vi "NanotecSMCPDDriver.get status.vi"(0 "VISA resource name":refnum<visa-resource-name>, 1 "contollerID":i32=-1, 5 "error in (no error)":errorcluster) -> (14 "VISA resource name out":refnum<visa-resource-name>, 15 "contollerID out":i32=-1, 17 "actStatus":T1, 19 "error out":errorcluster)   [LabVIEW 2015, in "NanotecSMCPDDriver.lvlib"]
doc: "Gets the status of the controller."
uses:
  NanotecSMCPDDriver.lvlib
  NanotecSMCPDDriver.status type.ctl
panel:
  in  "actStatus type":T1
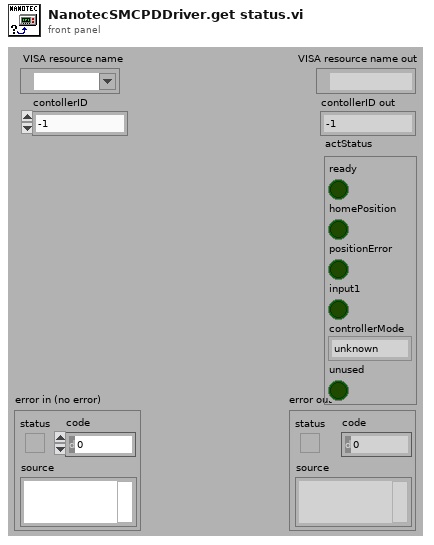
[diagram p1: front panel]
types:
  T1 = typedef "NanotecSMCPDDriver.lvlib/NanotecSMCPDDriver.status type.ctl" = cluster{"ready":bool, "homePosition":bool, "positionError":bool, "input1":bool, "controllerMode":enum16{"unknown", "position", "speed", "flagPosition", "clockDirection", "analog", "joystick", "unused"}, "unused":bool}
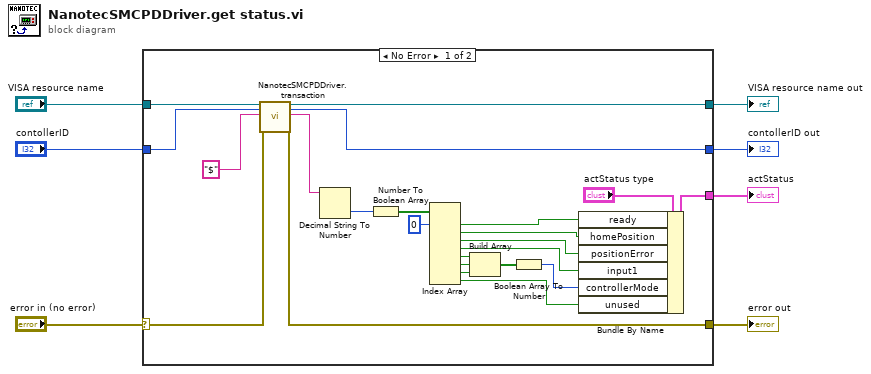
[diagram p0: block diagram]
diagram:
  n1 = case shown="No Error" "error in (no error)" {
    selector: "error in (no error)" -> [w23 w31]
    tunnel: [w26 w33] -> w7
    tunnel: [w24 w31] -> w6
    tunnel: "VISA resource name" -> [w30 w33]
    tunnel: "contollerID" -> [w28 w32]
    tunnel: [w27 w32] -> w3
    tunnel: [w8 _] -> w1
    frame No Error {
      n2 = call "NanotecSMCPDDriver.transaction.vi"("VISAresource"=w30, "contollerID"=w28, "commandString"="$", "error in (no error)"=w23) -> ("VISAresource out"=w26:refnum<visa-resource-name>, "contollerID out"=w27:i32, "response"=w25:string, "error out"=w24:errorcluster)  [unwired: 10 in, 2 out]
      n3 = Decimal String To Number(string=w25) -> (number=w22:i32)  [unwired: 2 in, 1 out]
      n4 = Number To Boolean Array(number=w22) -> (Boolean array=w21:bool[])
      n5 = Index Array(array=w21, index #1=0 ("index")) -> (element #1=w18:bool, element #2=w17:bool, element #3=w16:bool, element #4=w15:bool, element #5=w14:bool, element #6=w13:bool, element #7=w12:bool, element #8=w9:bool)  [unwired: 7 in]
      n6 = Build Array(w14, w13, w12) -> (w11:bool[])
      n7 = Boolean Array To Number(Boolean array=w11) -> (number=w10:u32)
      n8 = Bundle By Name(cluster="actStatus type", "ready"=w18, "homePosition"=w17, "positionError"=w16, "input1"=w15, "controllerMode"=w10, "unused"=w9) -> (w8:T1)
    }
    frame Error {
    }
  }
  "VISA resource name out" <- w7
  "error out" <- w6
  "contollerID out" <- w3
  "actStatus" <- w1
